vi "Basic_Acquire_Widefield.vi"() -> ()   [LabVIEW 2009]
uses:
  <vilib>/vision/Image Controls.llb/IMAQ Image.ctl
  <vilib>/userDefined/High Color/IMAQdx.ctl
  Widefield_globals.vi
  <vilib>/DAQmx/create/channels.llb/DAQmx Create Channel (DO-Digital Output).vi
  <vilib>/DAQmx/write.llb/DAQmx Write (Digital Bool 1Line 1Point).vi
  <vilib>/vision/NI_Vision_Development_Module.lvlib
  Program Files/National Instruments/LabVIEW 2009/resource/objmgr/imaqdx.rc
  <vilib>/vision/driver/NI_Vision_Acquisition_Software.lvlib
panel:
  out "RatioIm 2":u8[][](graph)
  out "frame number":i32
  out "IMAQ session":T1 caption="Session Out"
  out "frame times":i32[](array[numeric])
  out "error out":errorcluster
  out "LED settle":i32
  out "Control LED?":bool
  out "stim tag":string
  out "SF file":string
  out "One Bulb?":bool
  out "File Path":path
  out "SingleFrames":bool
  out "empty frame":dbl[][](array[numeric])
  out "Resolution":u32[](array[numeric])
  out "Experiment Sequence":dbl[][](array[numeric])
  out "settings":sgl[](array[numeric])
  out "Buff Img":T2
  out "COString":string
  in  "Offset (32768 default)":u32=32768
  in  "Contrast (600000 default)":u32=600000
  in  "Pause":bool=TRUE
  out "ExpOrderRefnum":refnum<file>
  out "Subframes":u32
  out "DCSAir":dbl[][](array[numeric])
  out "DCOdor":dbl[][](array[numeric])
  out "DCAir":dbl[][](array[numeric])
  out "TiffRefnum":refnum<file>
  out "Indices":i32[](array[numeric])
  out "Frames SAir":u32
  out "Odors:":u32
  out "StopAcq":bool
  in  "Stop":bool=TRUE
  out "Odor #":i32=50
  out "Repeats:":i32=1
  out "Repeat #":i32=1
  out "Frames Odor":u32
  out "Frames Air":u32
  out "Status":string
  out "Stimulus #":i32
  in  "start":bool=TRUE
  # "Filtered Ratio Image"
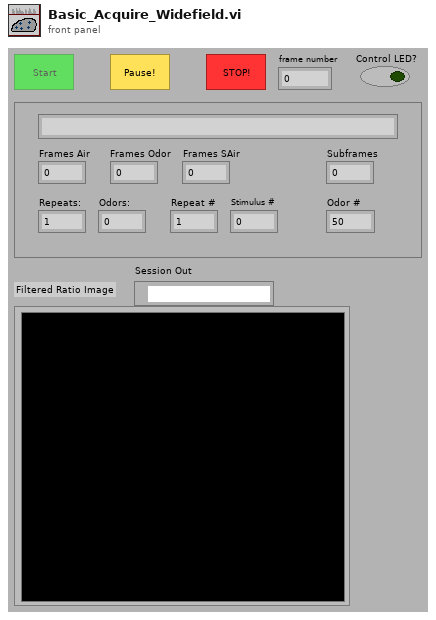
[diagram p1: front panel]
types:
  T1 = typedef "IMAQdx.ctl" = refnum<k21>
  T2 = typedef "IMAQ Image.ctl" = refnum<image>
  T3 = enum16{"open", "replace", "create", "open or create", "replace or create", "replace or create with confirmation"}
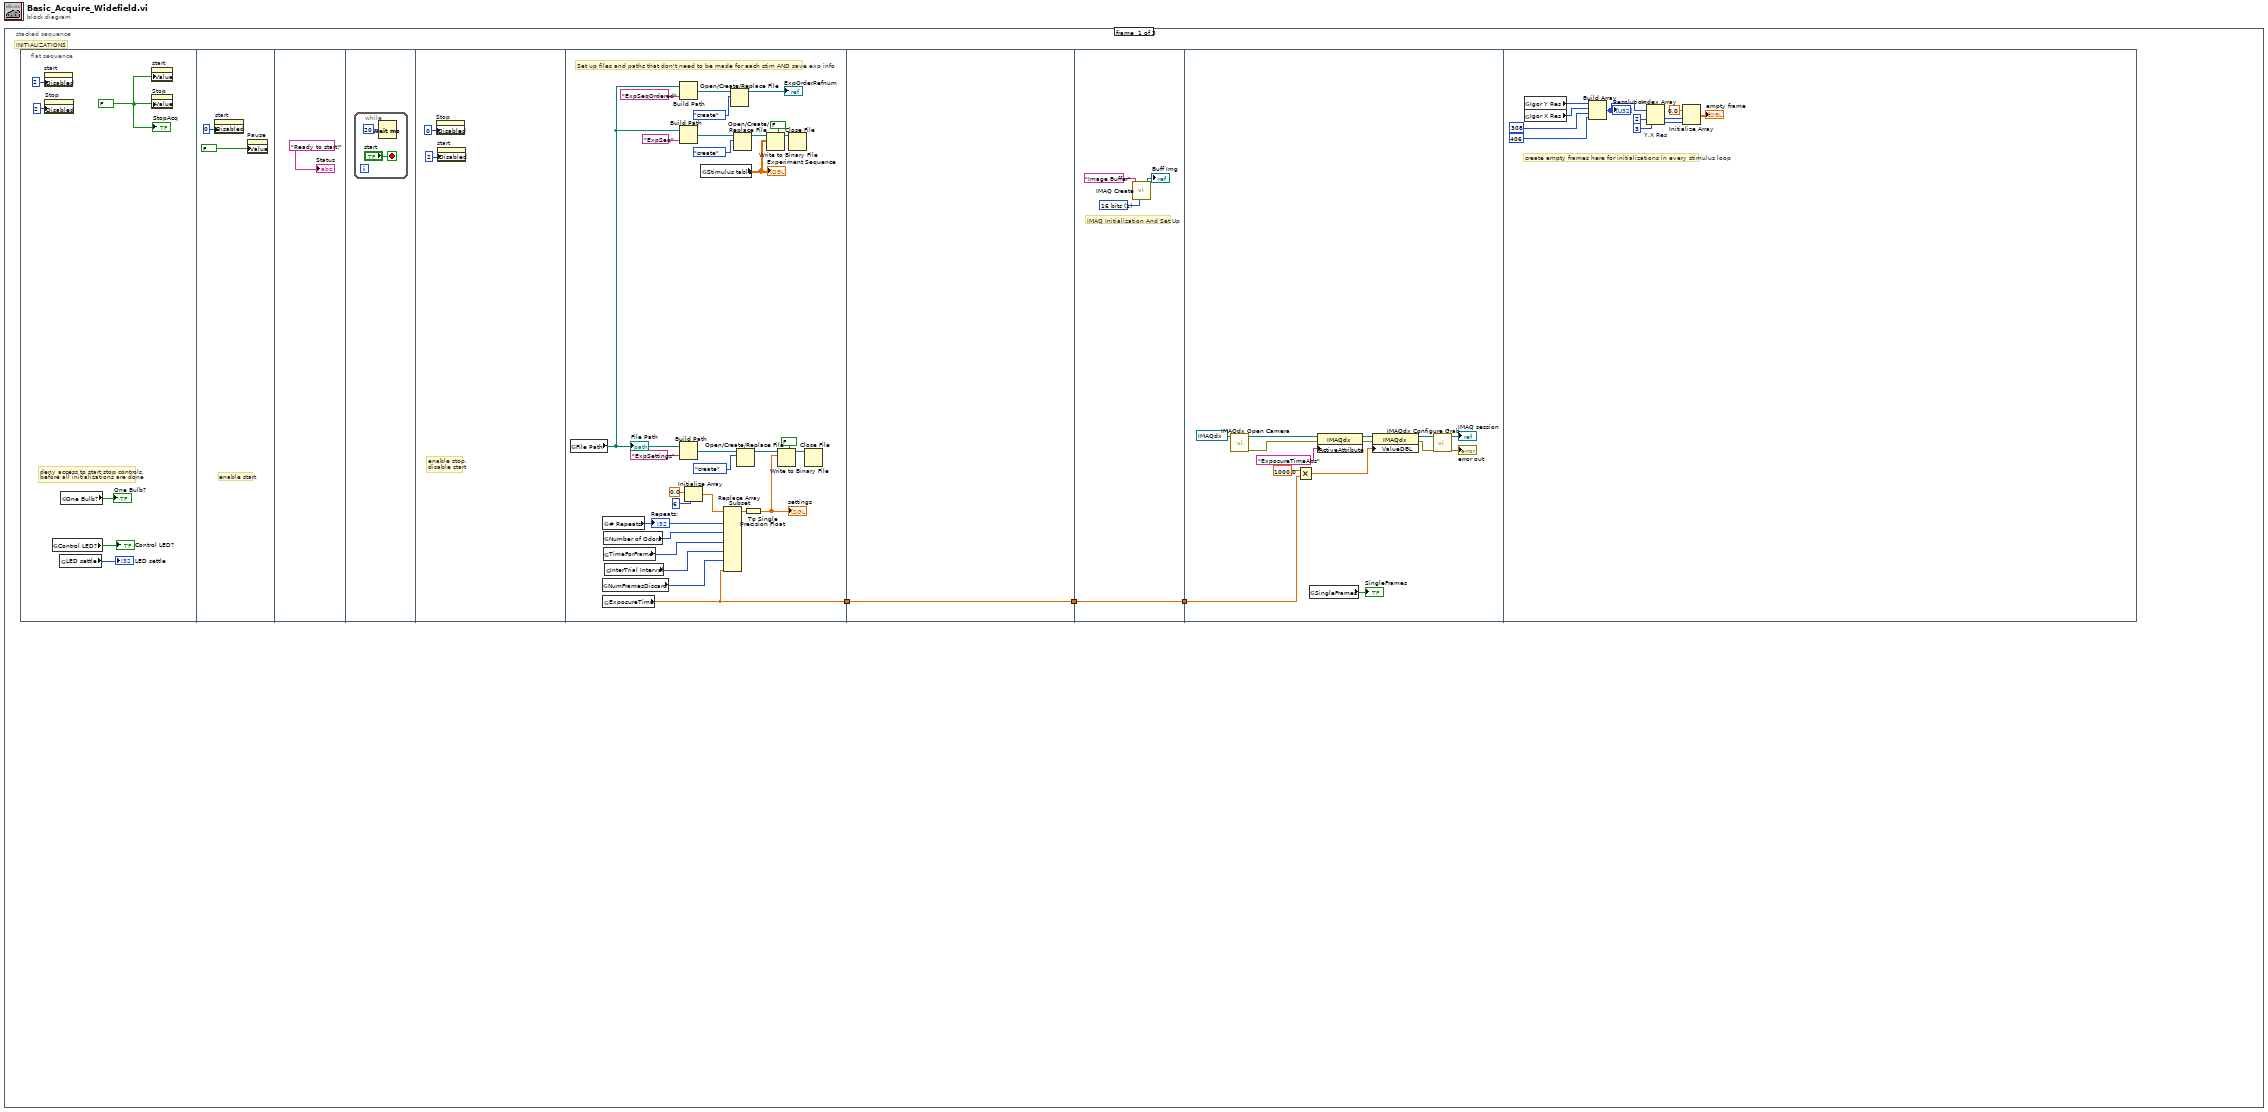
[diagram p0: block diagram]
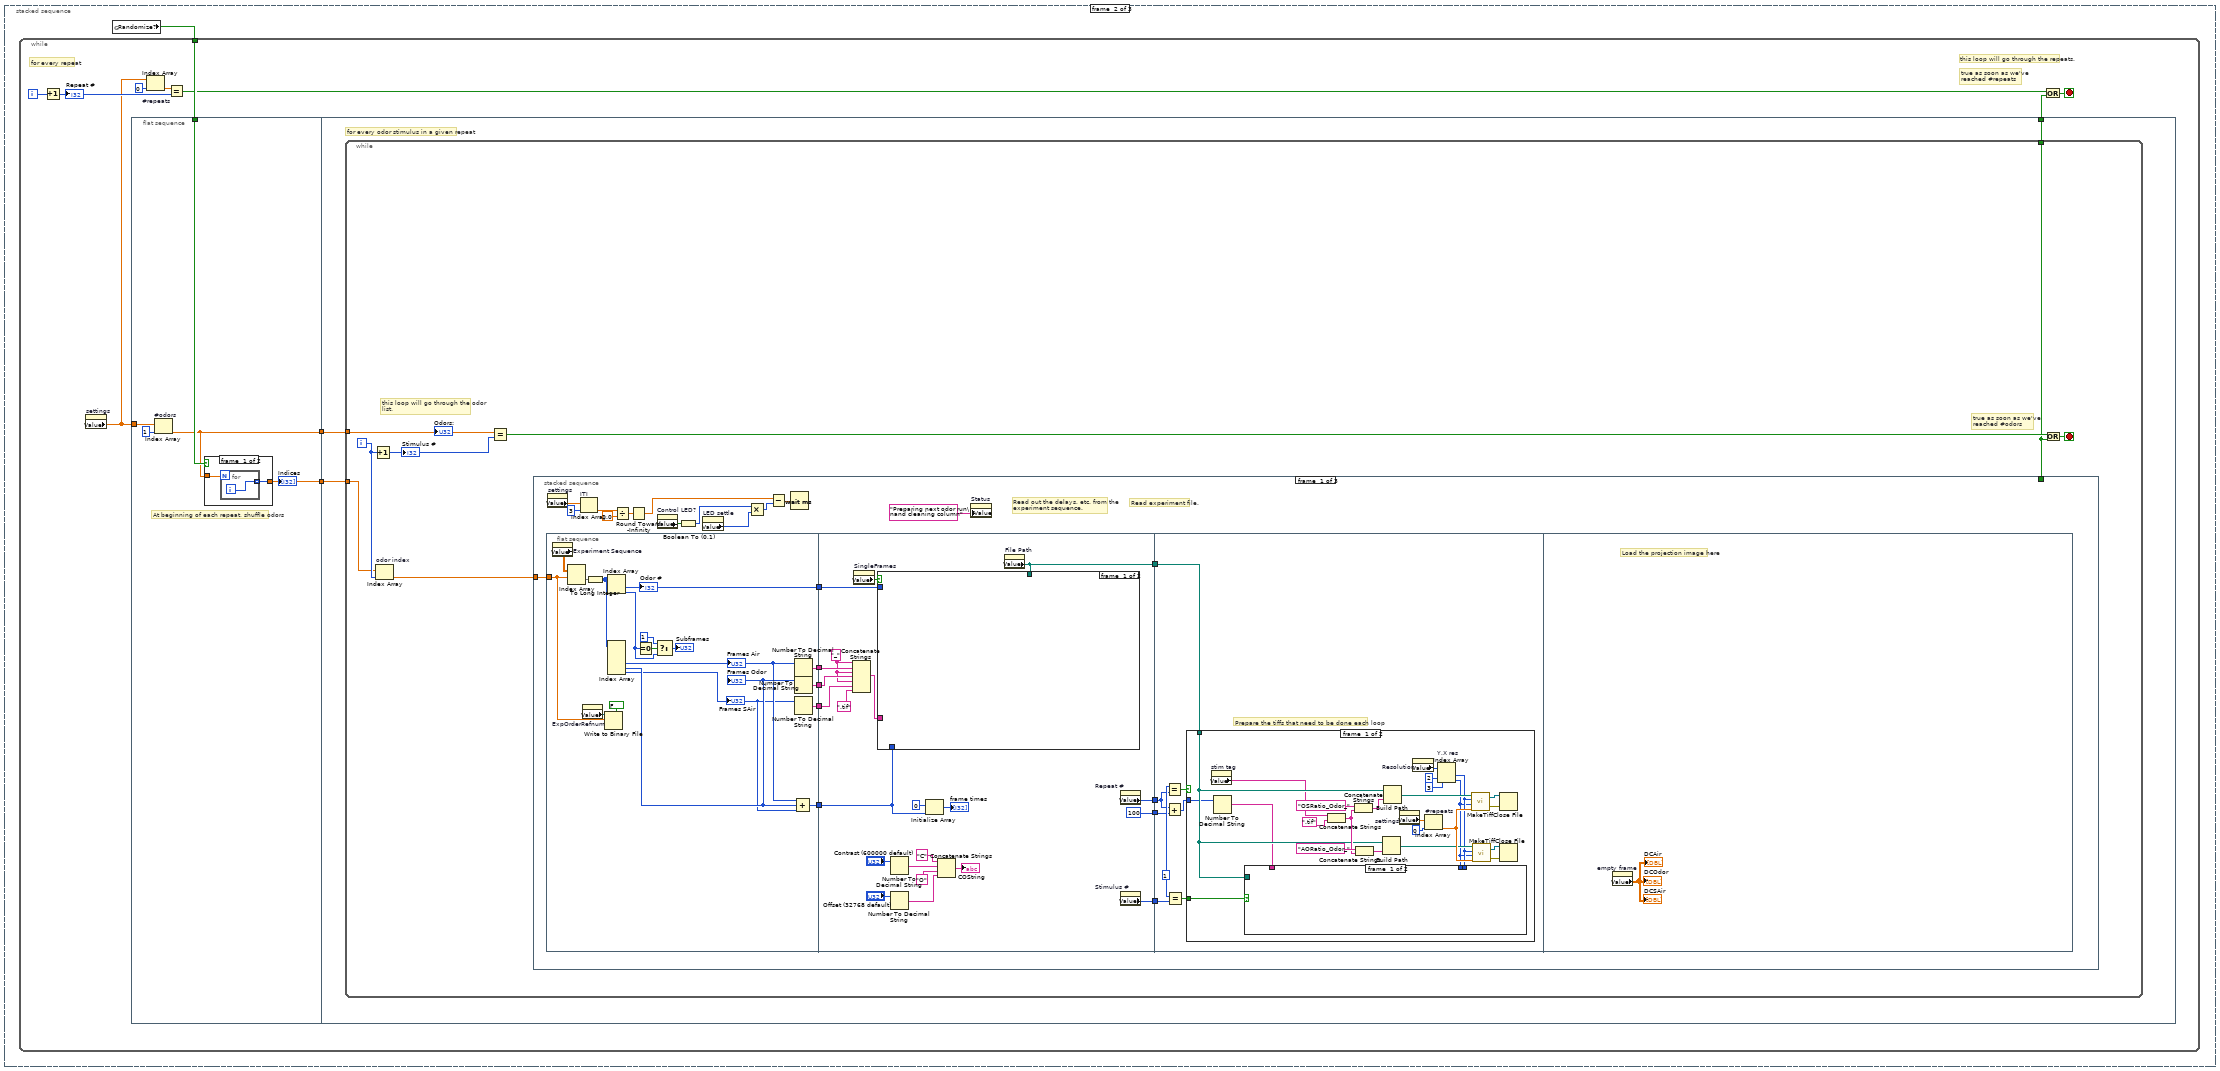
[diagram p2: hidden frame]
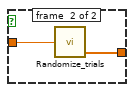
[diagram p3: hidden frame]
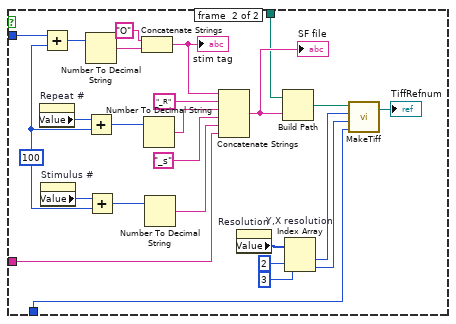
[diagram p4: hidden frame]
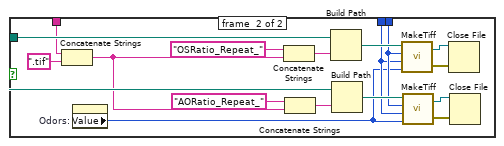
[diagram p5: hidden frame]
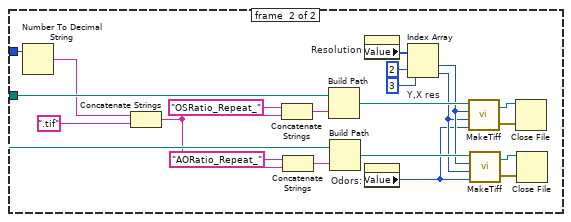
[diagram p7: hidden frame]
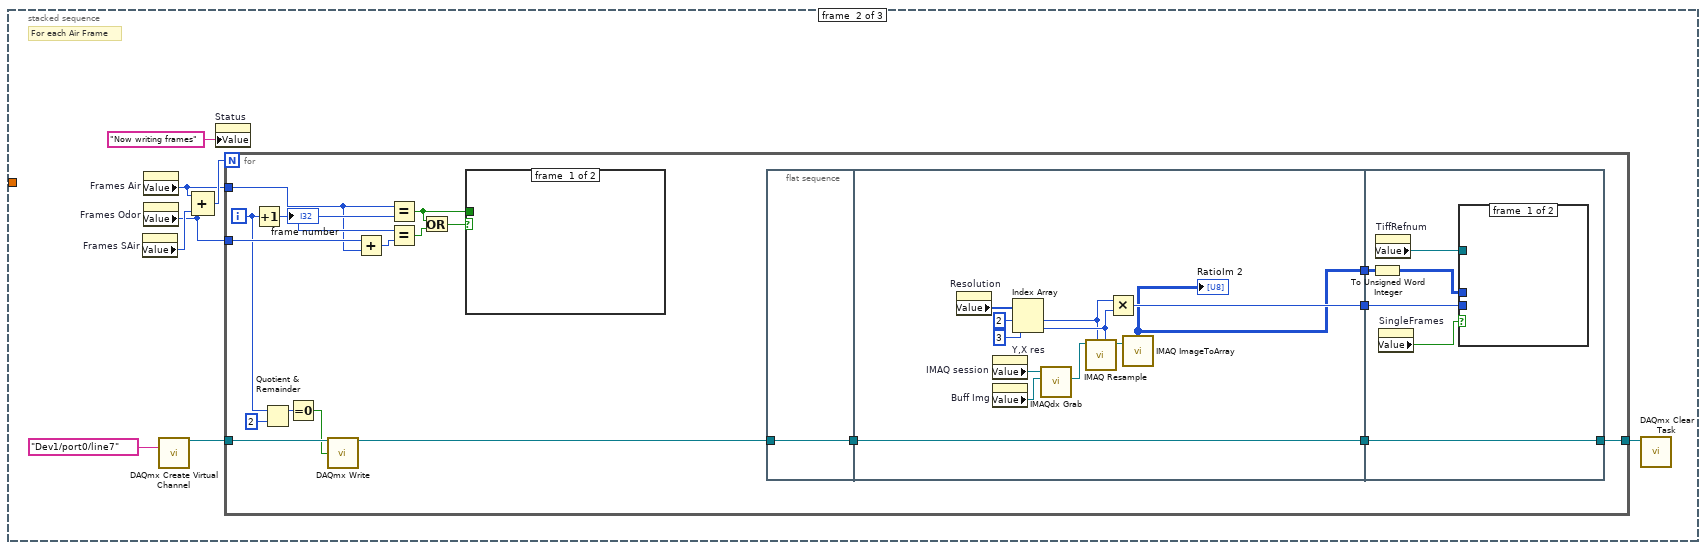
[diagram p8: hidden frame]
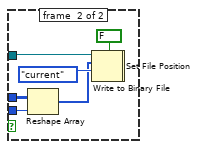
[diagram p9: hidden frame]
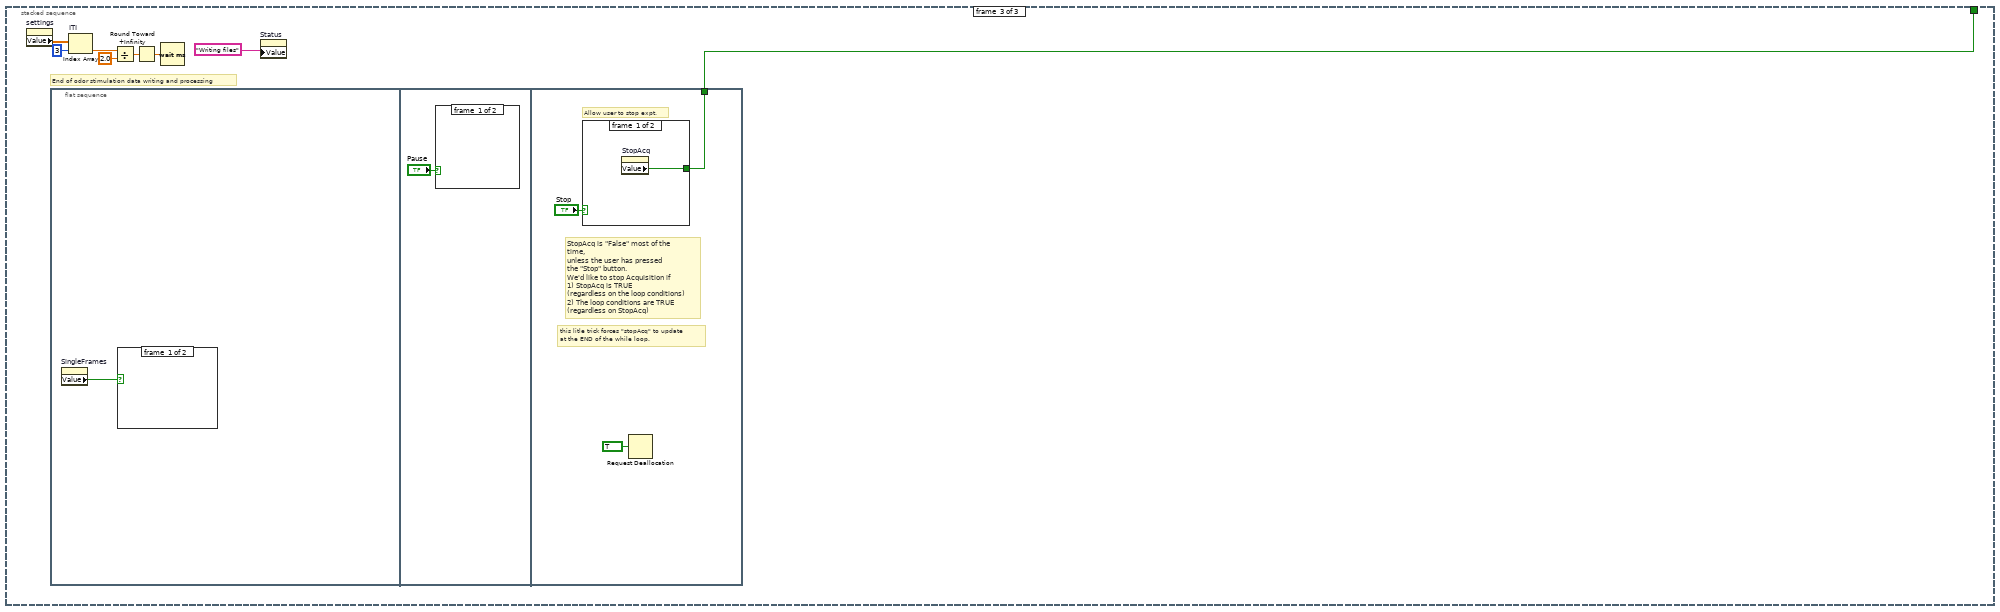
[diagram p12: hidden frame]
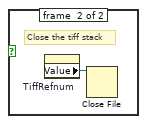
[diagram p13: hidden frame]
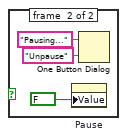
[diagram p14: hidden frame]
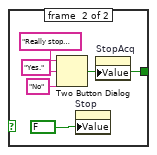
[diagram p15: hidden frame]
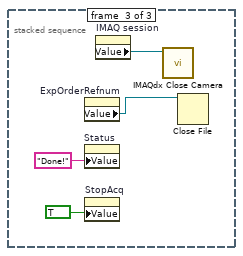
[diagram p16: hidden frame]
diagram:
  n1 = stacked-sequence {
    frame #0 {
      # "INITIALIZATIONS"
      n2 = flat-sequence {
        tunnel: [w18] -> w1
        tunnel: [w46] -> w2
        tunnel: w1 -> [w46]
        tunnel: [w47] -> w3
        tunnel: w2 -> [w47]
        tunnel: w3 -> [w57]
        frame #0 {
          w7 = FALSE ("Stop")
          # "deny access to start stop controls, \nbefore all initializations are done"
          n3 = property on="start" class="Boolean (strict)"("Disabled"=u8 2) -> ()  [unwired: 2 in, 2 out]
          n4 = property on="Stop" class="Bool (strict)"("Disabled"=u8 2) -> ()  [unwired: 2 in, 2 out]
          n5 = global read "Widefield_globals.vi" "Control LED?"() -> (→"Control LED?":bool)
          n6 = global read "Widefield_globals.vi" "LED settle"() -> (→"LED settle":i32)
          n7 = global read "Widefield_globals.vi" "One Bulb?"() -> (→"One Bulb?":bool)
          n8 = property on="start" class="Boolean (strict)"("Value"=w7) -> ()  [unwired: 2 in, 2 out]
          n9 = property on="Stop" class="Bool (strict)"("Value"=w7) -> ()  [unwired: 2 in, 2 out]
          "StopAcq" <- w7
        }
        frame #1 {
          # "enable start"
          n10 = property on="start" class="Boolean (strict)"("Disabled"=u8 0) -> ()  [unwired: 2 in, 2 out]
          n11 = property on="Pause" class="Bool (strict)"("Value"=FALSE ("Pause")) -> ()  [unwired: 2 in, 2 out]
        }
        frame #2 {
          "Status" <- "Ready to start!" ("Status")
        }
        frame #3 {
          n12 = while {
            stop <- "start" stop-if-true
            n13 = Wait (ms)(milliseconds to wait=u32 20) -> ()  [unwired: 1 out]
          }
        }
        frame #4 {
          # "enable stop,\ndisable start"
          n14 = property on="Stop" class="Bool (strict)"("Disabled"=u8 0) -> ()  [unwired: 2 in, 2 out]
          n15 = property on="start" class="Boolean (strict)"("Disabled"=u8 2) -> ()  [unwired: 2 in, 2 out]
        }
        frame #5 {
          # "Set up files and paths that don't need to be made for each stim AND save exp info"
          n16 = global read "Widefield_globals.vi" "File Path"() -> (w24:path)
          "File Path" <- w24
          n17 = global read "Widefield_globals.vi" "NumFramesDiscard"() -> (w19:i32)
          n18 = global read "Widefield_globals.vi" "# Repeats"() -> (w22:u16)
          "Repeats:" <- w22
          n19 = global read "Widefield_globals.vi" "ExposureTime"() -> (w18:dbl)
          n20 = global read "Widefield_globals.vi" "Number of Odors"() -> (w21:u32)
          n21 = global read "Widefield_globals.vi" "TimeForFrame"() -> (w17:u32)
          n22 = global read "Widefield_globals.vi" "InterTrial Interval"() -> (w20:i32)
          n23 = Build Path(base path=w24, name or relative path="ExpSeq" ("string")) -> (appended path=w37:path)
          n24 = Build Path(base path=w24, name or relative path="ExpSeqOrdered" ("string")) -> (appended path=w27:path)
          n25 = Build Path(base path=w24, name or relative path="ExpSettings" ("string")) -> (appended path=w35:path)
          n26 = Initialize Array(sgl 0.0 ("element"), 6 ("dimension size")) -> (w31:sgl[])
          n27 = global read "Widefield_globals.vi" "Stimulus table"() -> (w23:dbl[][])
          "Experiment Sequence" <- w23
          n28 = Replace Array Subset(array=w31, new element #1=w22, new element #2=w21, new element #3=w17, new element #4=w20, new element #5=w19, new element #6=w18) -> (w30:sgl[])  [unwired: 6 in]
          n29 = Open/Create/Replace File(file path (use dialog)=w27, operation (0:open)=T3."create") -> (refnum out=→"ExpOrderRefnum":refnum<file>)  [unwired: 1 in, 5 out]
          n30 = Open/Create/Replace File(file path (use dialog)=w37, operation (0:open)=T3."create") -> (refnum out=w44:refnum<file>)  [unwired: 1 in, 5 out]
          n31 = Open/Create/Replace File(file path (use dialog)=w35, operation (0:open)=T3."create") -> (refnum out=w43:refnum<file>)  [unwired: 1 in, 5 out]
          n32 = To Single Precision Float(number=w30) -> (single precision float=w29:sgl[])
          "settings" <- w29
          n33 = Write to Binary File(file (use dialog)=w44, data=w23, 5:FALSE ("prepend array or string size? (T)")) -> (refnum out=w45:refnum<file>)  [unwired: 1 in, 4 out]
          n34 = Write to Binary File(file (use dialog)=w43, data=w29, 5:FALSE ("prepend array or string size? (T)")) -> (refnum out=w28:refnum<file>)  [unwired: 1 in, 4 out]
          n35 = Close File(refnum=w45) -> ()  [unwired: 1 in, 2 out]
          n36 = Close File(refnum=w28) -> ()  [unwired: 1 in, 2 out]
        }
        frame #6 {
        }
        frame #7 {
          w50 = u32 1 items=["8 bits", "16 bits", "Float", "Complex", "RGB", "HSL"] ("Image Type")
          # "IMAQ Initialization And Set Up"
          n37 = call "IMAQ Create"("Image Name"="Image Buffer", "Image Type"=w50) -> ("New Image"=→"Buff Img":T2)  [unwired: 2 in, 2 out]
        }
        frame #8 {
          n38 = call <vilib>:"IMAQdx Open Camera.vi"("Session In"=T1 "cam0") -> ("error out"=w60:errorcluster, "Session Out"=w59:T1)  [unwired: 2 in, 7 out]
          n39 = Multiply(x=1000.0 ("y"), y=w57) -> (x*y=w53:dbl)
          n40 = global read "Widefield_globals.vi" "SingleFrames"() -> (→"SingleFrames":bool)
          n41 = property class="IMAQdx"(reference=w59, error in=w60, "ActiveAttribute"="ExposureTimeAbs" ("Camera Attribute")) -> (reference out=w54:T1, error out=w55:errorcluster)
          n42 = property class="IMAQdx"(reference=w54, error in=w55, "ValueDBL"=w53) -> (reference out=w62:T1, error out=w58:errorcluster)
          n43 = call <vilib>:"IMAQdx Configure Grab.vi"("error in"=w58, "Session In"=w62) -> ("error out"=→"error out":errorcluster, "Session Out"=→"IMAQ session":T1)  [unwired: 8 out]
        }
        frame #9 {
          # "create empty frames here for initializations in every stimulus loop"
          n44 = global read "Widefield_globals.vi" "Igor Y Res"() -> (w69:u32)
          n45 = global read "Widefield_globals.vi" "Igor X Res"() -> (w68:u32)
          n46 = Build Array(w69, w68, u32 308 ("Y Res"), u32 406 ("X Res")) -> (w67:u32[])
          "Resolution" <- w67
          n47 = Index Array "Y,X Res"(array=w67, index #1=2 ("index"), index #2=3 ("index")) -> (element #1=w75:u32, element #2=w74:u32)
          n48 = Initialize Array(0.0 ("element"), w75, w74) -> (→"empty frame":dbl[][])
        }
      }
    }
    frame #1 {
      n49 = global read "Widefield_globals.vi" "Randomize?"() -> (w76:bool)
      n50 = while {
        tunnel: w76 -> [w85]
        i -> [w80]
        stop <- w87 stop-if-true
        # "for every repeat"
        # "this loop will go through the repeats."
        # "true as soon as we've\nreached #repeats"
        n51 = Increment(x=w80) -> (x+1=w86:i32)
        "Repeat #" <- w86
        n52 = property on="settings" class="Arr (strict)"() -> ("Value"=w82:sgl[])  [unwired: 2 in, 2 out]
        n53 = flat-sequence {
          tunnel: w82 -> [w92]
          tunnel: w85 -> [w90]
          tunnel: [w89] -> w84
          tunnel: [w88] -> w83
          tunnel: w84 -> [w100]
          tunnel: w83 -> [w99]
          tunnel: [w98] -> w78
          frame #0 {
            # "At beginning of each repeat, shuffle odors"
            n54 = Index Array "#odors"(array=w92, index=1) -> (element=w89:sgl)
            n55 = case shown="True" w90 {
              tunnel: [w93 w97] -> w88
              tunnel: w89 -> [w94 w96]
              frame #0 {
                n56 = for {
                  N: w94 -> [_]
                  tunnel: [w95] -> w93 mode=indexing
                  i -> [w95]
                }
              }
              frame #1 {
                n57 = call "Randomize_trials.vi"("ArraySize"=w96) -> ("Randomized"=w97:dbl[])  [unwired: 2 in]
              }
            }
            "Indices" <- w88
          }
          frame #1 {
            # "for every odor stimulus in a given repeat"
            n58 = while {
              tunnel: w100 -> [w107]
              tunnel: w99 -> [w104]
              tunnel: [w102] -> w98
              i -> [w106]
              stop <- w108 stop-if-true
              # "this loop will go through the odor\nlist."
              # "true as soon as we've\nreached #odors"
              n59 = Increment(x=w106) -> (x+1=w101:i32)
              "Stimulus #" <- w101
              n60 = Index Array "odor index"(array=w104, index=w106) -> (element=w105:dbl)
              n61 = Equal?(x=w107, y=w101) -> (x = y?=w103:bool)
              n62 = stacked-sequence {
                tunnel: w105 -> [w130 _ _]
                tunnel: [_ _ w332] -> w102
                frame #0 {
                  # "Read experiment file."
                  # "Read out the delays, etc. from the\nexperiment sequence."
                  n63 = flat-sequence {
                    tunnel: [w146] -> w129
                    tunnel: [w145] -> w128
                    tunnel: [w144] -> w127
                    tunnel: [w143] -> w126
                    tunnel: [w142] -> w125
                    tunnel: w130 -> [w134]
                    tunnel: [w162] -> w124
                    tunnel: [w163] -> w123
                    tunnel: [w161] -> w122
                    tunnel: w125 -> [w151]
                    tunnel: w126 -> [w157]
                    tunnel: w127 -> [w158]
                    tunnel: w128 -> [w159]
                    tunnel: w129 -> [w160]
                    tunnel: [100 ("y")] -> w114
                    tunnel: w124 -> [w197]
                    tunnel: w123 -> [w202]
                    tunnel: w122 -> [w201]
                    tunnel: w114 -> [w198]
                    frame #0 {
                      n64 = property on="Experiment Sequence" class="Arr (strict)"() -> ("Value"=w141:dbl[][])  [unwired: 2 in, 2 out]
                      n65 = Index Array(array=w141, index (row)=w134) -> (element=w140:dbl[])  [unwired: 1 in]
                      n66 = property on="ExpOrderRefnum" class="Ref (strict)"() -> ("Value"=w147:refnum<file>)  [unwired: 2 in, 2 out]
                      n67 = To Long Integer(number=w140) -> (32bit integer=w136:i32[])
                      n68 = Write to Binary File(file (use dialog)=w147, data=w134, 5:FALSE ("prepend array or string size? (T)")) -> ()  [unwired: 1 in, 5 out]
                      n69 = Index Array(array=w136) -> (element #1=w143:i32, element #2=w133:i32)  [unwired: 2 in]
                      "Odor #" <- w143
                      n70 = Index Array(array=w136) -> (element #3=w132:i32, element #4=w135:i32, element #5=w131:i32)  [unwired: 5 in, 2 out]
                      "Frames Air" <- w132
                      "Frames Odor" <- w135
                      "Frames SAir" <- w131
                      n71 = Equal To 0?(x=w133) -> (x = 0?=w139:bool)
                      n72 = Select(t=1, s=w139, f=w133) -> (s? t:f=→"Subframes":i32)
                      n73 = Number To Decimal String(number=w132) -> (decimal integer string=w146:string)  [unwired: 1 out]
                      n74 = Number To Decimal String(number=w135) -> (decimal integer string=w145:string)  [unwired: 1 out]
                      n75 = Number To Decimal String(number=w131) -> (decimal integer string=w144:string)  [unwired: 1 out]
                      n76 = Compound Arithmetic op=ADD(w132, w135, w131) -> (w142:i32)
                    }
                    frame #1 {
                      w154 = "_" ("string")
                      n77 = Concatenate Strings(w154, w160, w154, w159, w154, w158, ".tif" ("string")) -> (w155:string)
                      n78 = property on="SingleFrames" class="Bool (strict)"() -> ("Value"=w156:bool)  [unwired: 2 in, 2 out]
                      n79 = Number To Decimal String(number="Contrast (600000 default)") -> (decimal integer string=w166:string)  [unwired: 1 out]
                      n80 = Number To Decimal String(number="Offset (32768 default)") -> (decimal integer string=w165:string)  [unwired: 1 out]
                      n81 = Initialize Array(0 ("element"), w151) -> (→"frame times":i32[])
                      n82 = Concatenate Strings("C" ("string"), w166, "O" ("string"), w165) -> (→"COString":string)
                      n83 = property on="File Path" class="Path"() -> ("Value"=w163:path)  [unwired: 2 in, 2 out]
                      n84 = case shown="True" w156 {
                        tunnel: w157 -> [_ w190]
                        tunnel: w163 -> [_ w178]
                        tunnel: w155 -> [_ w171]
                        tunnel: w151 -> [_ w188]
                        frame #0 {
                        }
                        frame #1 {
                          w189 = 100 ("y")
                          n85 = property on="Repeat #" class="DigNum (strict)"() -> ("Value"=w181:i32)  [unwired: 2 in, 2 out]
                          n86 = property on="Stimulus #" class="DigNum (strict)"() -> ("Value"=w174:i32)  [unwired: 2 in, 2 out]
                          n87 = Add(x=w190, y=w189) -> (x+y=w194:i32)
                          n88 = Number To Decimal String(number=w194) -> (decimal integer string=w176:string)  [unwired: 1 out]
                          n89 = Add(x=w181, y=w189) -> (x+y=w195:i32)
                          n90 = Add(x=w174, y=w189) -> (x+y=w191:i32)
                          n91 = Concatenate Strings("O" ("string"), w176) -> (w175:string)
                          "stim tag" <- w175
                          n92 = Number To Decimal String(number=w195) -> (decimal integer string=w193:string)  [unwired: 1 out]
                          n93 = Number To Decimal String(number=w191) -> (decimal integer string=w172:string)  [unwired: 1 out]
                          n94 = Concatenate Strings(w175, "_R" ("string"), w193, "_s" ("string"), w172, w171) -> (w180:string)
                          "SF file" <- w180
                          n95 = property on="Resolution" class="Arr (strict)"() -> ("Value"=w186:u32[])  [unwired: 2 in, 2 out]
                          n96 = Build Path(base path=w178, name or relative path=w180) -> (appended path=w179:path)
                          n97 = Index Array "Y,X resolution"(array=w186, index #1=2 ("index"), index #2=3 ("index")) -> (element #1=w183:u32, element #2=w182:u32)
                          n98 = call "MakeTiff.vi"("z"=w188, "X"=w182, "Y"=w183, "file path"=w179) -> ("refnum tif"=→"TiffRefnum":refnum<file>)  [unwired: 1 out]
                        }
                      }
                      n99 = property on="Repeat #" class="DigNum (strict)"() -> ("Value"=w162:i32)  [unwired: 2 in, 2 out]
                      n100 = property on="Stimulus #" class="DigNum (strict)"() -> ("Value"=w161:i32)  [unwired: 2 in, 2 out]
                    }
                    frame #2 {
                      w200 = 1 ("x")
                      # "Prepare the tiffs that need to be done each loop"
                      n101 = Equal?(x=w200, y=w197) -> (x = y?=w203:bool)
                      n102 = Add(x=w197, y=w198) -> (x+y=w196:i32)
                      n103 = Equal?(x=w200, y=w201) -> (x = y?=w199:bool)
                      n104 = case shown="False" w203 {
                        tunnel: w202 -> [w211 w248]
                        tunnel: w196 -> [w207 w247]
                        tunnel: w199 -> [w206 w246]
                        frame #0 {
                          n105 = property on="stim tag" class="Str"() -> ("Value"=w205:string)  [unwired: 2 in, 2 out]
                          n106 = Number To Decimal String(number=w207) -> (decimal integer string=w208:string)  [unwired: 1 out]
                          n107 = Concatenate Strings(w205, ".tif" ("string")) -> (w220:string)
                          n108 = Concatenate Strings("OSRatio_Odor_" ("string"), w220) -> (w222:string)
                          n109 = Concatenate Strings("AORatio_Odor_" ("string"), w220) -> (w219:string)
                          n110 = Build Path(base path=w211, name or relative path=w219) -> (appended path=w212:path)
                          n111 = Build Path(base path=w211, name or relative path=w222) -> (appended path=w224:path)
                          n112 = property on="settings" class="Arr (strict)"() -> ("Value"=w214:sgl[])  [unwired: 2 in, 2 out]
                          n113 = property on="Resolution" class="Arr (strict)"() -> ("Value"=w218:u32[])  [unwired: 2 in, 2 out]
                          n114 = Index Array "#repeats"(array=w214, index=0) -> (element=w213:sgl)
                          n115 = Index Array "Y,X res"(array=w218, index #1=2 ("index"), index #2=3 ("index")) -> (element #1=w210:u32, element #2=w209:u32)
                          n116 = case shown="True" w206 {
                            tunnel: w211 -> [_ w235]
                            tunnel: w210 -> [_ w234]
                            tunnel: w209 -> [_ w233]
                            tunnel: w208 -> [_ w231]
                            frame #0 {
                            }
                            frame #1 {
                              n117 = Concatenate Strings(w231, ".tif" ("string")) -> (w232:string)
                              n118 = property on="Odors:" class="DigNum (strict)"() -> ("Value"=w230:u32)  [unwired: 2 in, 2 out]
                              n119 = Concatenate Strings("OSRatio_Repeat_" ("string"), w232) -> (w245:string)
                              n120 = Concatenate Strings("AORatio_Repeat_" ("string"), w232) -> (w237:string)
                              n121 = Build Path(base path=w235, name or relative path=w245) -> (appended path=w236:path)
                              n122 = Build Path(base path=w235, name or relative path=w237) -> (appended path=w239:path)
                              n123 = call "MakeTiff.vi"("z"=w230, "X"=w233, "Y"=w234, "file path"=w236) -> ("error out"=w243:errorcluster, "refnum tif"=w242:refnum<file>)
                              n124 = call "MakeTiff.vi"("z"=w230, "X"=w233, "Y"=w234, "file path"=w239) -> ("error out"=w240:errorcluster, "refnum tif"=w241:refnum<file>)
                              n125 = Close File(refnum=w242, error in=w243) -> ()  [unwired: 2 out]
                              n126 = Close File(refnum=w241, error in=w240) -> ()  [unwired: 2 out]
                            }
                          }
                          n127 = call "MakeTiff.vi"("z"=w213, "X"=w209, "Y"=w210, "file path"=w224) -> ("error out"=w225:errorcluster, "refnum tif"=w226:refnum<file>)
                          n128 = call "MakeTiff.vi"("z"=w213, "X"=w209, "Y"=w210, "file path"=w212) -> ("error out"=w227:errorcluster, "refnum tif"=w228:refnum<file>)
                          n129 = Close File(refnum=w226, error in=w225) -> ()  [unwired: 2 out]
                          n130 = Close File(refnum=w228, error in=w227) -> ()  [unwired: 2 out]
                        }
                        frame #1 {
                          n131 = case shown="True" w246 {
                            tunnel: w248 -> [_ w256]
                            tunnel: w247 -> [_ w251]
                            frame #0 {
                            }
                            frame #1 {
                              n132 = Number To Decimal String(number=w251) -> (decimal integer string=w252:string)  [unwired: 1 out]
                              n133 = Concatenate Strings(w252, ".tif" ("string")) -> (w253:string)
                              n134 = Concatenate Strings("OSRatio_Repeat_" ("string"), w253) -> (w266:string)
                              n135 = Concatenate Strings("AORatio_Repeat_" ("string"), w253) -> (w258:string)
                              n136 = Build Path(base path=w256, name or relative path=w266) -> (appended path=w257:path)
                              n137 = Build Path(base path=w256, name or relative path=w258) -> (appended path=w260:path)
                              n138 = property on="Resolution" class="Arr (strict)"() -> ("Value"=w269:u32[])  [unwired: 2 in, 2 out]
                              n139 = property on="Odors:" class="DigNum (strict)"() -> ("Value"=w250:u32)  [unwired: 2 in, 2 out]
                              n140 = Index Array "Y,X res"(array=w269, index #1=2 ("index"), index #2=3 ("index")) -> (element #1=w255:u32, element #2=w254:u32)
                              n141 = call "MakeTiff.vi"("z"=w250, "X"=w254, "Y"=w255, "file path"=w257) -> ("error out"=w264:errorcluster, "refnum tif"=w263:refnum<file>)
                              n142 = call "MakeTiff.vi"("z"=w250, "X"=w254, "Y"=w255, "file path"=w260) -> ("error out"=w261:errorcluster, "refnum tif"=w262:refnum<file>)
                              n143 = Close File(refnum=w263, error in=w264) -> ()  [unwired: 2 out]
                              n144 = Close File(refnum=w262, error in=w261) -> ()  [unwired: 2 out]
                            }
                          }
                        }
                      }
                    }
                    frame #3 {
                      # "Load the projection image here"
                      n145 = property on="empty frame" class="Arr (strict)"() -> ("Value"=→"DCAir" →"DCOdor" →"DCSAir":dbl[][])  [unwired: 2 in, 2 out]
                    }
                  }
                  n146 = property on="settings" class="Arr (strict)"() -> ("Value"=w121:sgl[])  [unwired: 2 in, 2 out]
                  n147 = Index Array "ITI"(array=w121, index=3) -> (element=w119:sgl)
                  n148 = Divide(x=w119, y=sgl 2.0) -> (x/y=w117:sgl)
                  n149 = Round Toward -Infinity(1:w117) -> (0:w116:sgl)
                  n150 = property on="Control LED?" class="Bool (strict)"() -> ("Value"=w112:bool)  [unwired: 2 in, 2 out]
                  n151 = Boolean To (0,1)(Boolean=w112) -> (0, 1=w110:i16)
                  n152 = property on="LED settle" class="DigNum (strict)"() -> ("Value"=w109:i32)  [unwired: 2 in, 2 out]
                  n153 = Multiply(x=w110, y=w109) -> (x*y=w111:i32)
                  n154 = Subtract(x=w116, y=w111) -> (x-y=w113:sgl)
                  n155 = Wait (ms)(milliseconds to wait=w113) -> ()  [unwired: 1 out]
                  n156 = property on="Status" class="Str"("Value"="Preparing next odor run\nand cleaning column" ("Status")) -> ()  [unwired: 2 in, 2 out]
                }
                frame #1 {
                  # "For each Air Frame"
                  n157 = property on="Frames SAir" class="DigNum (strict)"() -> ("Value"=w277:u32)  [unwired: 2 in, 2 out]
                  n158 = property on="Frames Air" class="DigNum (strict)"() -> ("Value"=w275:u32)  [unwired: 2 in, 2 out]
                  n159 = property on="Frames Odor" class="DigNum (strict)"() -> ("Value"=w274:u32)  [unwired: 2 in, 2 out]
                  n160 = call-poly <vilib>:"DAQmx Create Virtual Channel.vi"("lines"=tag "Dev1/port0/line7") -> ("task out"=w272:refnum<k21>)  [unwired: 13 in, 1 out]
                  n161 = Compound Arithmetic op=ADD(w275, w274, w277) -> (w276:u32)
                  n162 = property on="Status" class="Str"("Value"="Now writing frames" ("String")) -> ()  [unwired: 2 in, 2 out]
                  n163 = for {
                    N: w276 -> [_]
                    tunnel: w275 -> [w291]
                    tunnel: w274 -> [w293]
                    tunnel: w272 -> [w284]
                    tunnel: [w279] -> w271
                    i -> [w287]
                    n164 = Increment(x=w287) -> (x+1=w294:i32)
                    "frame number" <- w294
                    n165 = Quotient & Remainder(x=w287, y=2) -> (x-y*floor(x/y)=w285:i32)  [unwired: 1 out]
                    n166 = Equal To 0?(x=w285) -> (x = 0?=w283:bool)
                    n167 = call-poly <vilib>:"DAQmx Write.vi"("task/channels in"=w284, "data"=w283) -> ("task out"=w280:refnum<k21>)  [unwired: 11 in, 2 out]
                    n168 = Add(x=w293, y=w291) -> (x+y=w292:u32)
                    n169 = Equal?(x=w291, y=w294) -> (x = y?=w288:bool)
                    n170 = Equal?(x=w294, y=w292) -> (x = y?=w289:bool)
                    n171 = Or(x=w288, y=w289) -> (x .or. y?=w290:bool)
                    n172 = case shown="True" w290 {
                      tunnel: w288 -> [_ w324]
                      frame #0 {
                      }
                      frame #1 {
                        n173 = case shown="True" w324 {
                          frame #0 {
                          }
                          frame #1 {
                          }
                        }
                      }
                    }
                    n174 = flat-sequence {
                      tunnel: [w297] -> w281
                      tunnel: w280 -> [w297]
                      tunnel: [w309] -> w296
                      tunnel: [w299] -> w295
                      tunnel: [w298] -> w282
                      tunnel: w281 -> [w298]
                      tunnel: w296 -> [w315]
                      tunnel: w295 -> [w314]
                      tunnel: w282 -> [w310]
                      tunnel: [w310] -> w279
                      frame #0 {
                      }
                      frame #1 {
                        n175 = property on="Resolution" class="Arr (strict)"() -> ("Value"=w306:u32[])  [unwired: 2 in, 2 out]
                        n176 = property on="IMAQ session" class="IMAQdx (strict)"() -> ("Value"=w304:refnum<k21>)  [unwired: 2 in, 2 out]
                        n177 = property on="Buff Img" class="IMAQImage (strict)"() -> ("Value"=w305:refnum<image>)  [unwired: 2 in, 2 out]
                        n178 = Index Array "Y,X res"(array=w306, index #1=2 ("index"), index #2=3 ("index")) -> (element #1=w302:u32, element #2=w303:u32)
                        n179 = call <vilib>:"IMAQdx Grab.vi"("Image In"=w305, "Session In"=w304) -> ("Image Out"=w301:T2)  [unwired: 2 in, 7 out]
                        n180 = call "IMAQ Resample"("X Resolution"=w303, "Y Resolution"=w302, "Image Src"=w301) -> ("Image Dst Out"=w300:T2)  [unwired: 4 in, 4 out]
                        n181 = Multiply(x=w302, y=w303) -> (x*y=w309:u32)
                        n182 = call "IMAQ ImageToArray"("Image"=w300) -> ("Image Pixels (U8)"=w299:u8[][])  [unwired: 2 in, 5 out]
                        "RatioIm 2" <- w299
                      }
                      frame #2 {
                        n183 = To Unsigned Word Integer(number=w314) -> (unsigned 16bit integer=w313:u16[][])
                        n184 = property on="TiffRefnum" class="Ref (strict)"() -> ("Value"=w312:refnum<file>)  [unwired: 2 in, 2 out]
                        n185 = property on="SingleFrames" class="Bool (strict)"() -> ("Value"=w311:bool)  [unwired: 2 in, 2 out]
                        n186 = case shown="True" w311 {
                          tunnel: w315 -> [_ w322]
                          tunnel: w313 -> [_ w320]
                          tunnel: w312 -> [_ w319]
                          frame #0 {
                          }
                          frame #1 {
                            n187 = Reshape Array(w320, w322) -> (w321:u16[])
                            n188 = Set File Position(refnum=w319, from (0:start)=enum16{"start", "end", "current"}."current" ("pos mode (0:2)")) -> (refnum out=w318:refnum<file>, error out=w317:errorcluster)  [unwired: 1 in, 1 out]
                            n189 = Write to Binary File(file (use dialog)=w318, data=w321, error in=w317, 5:FALSE ("prepend array or string size? (T)")) -> ()  [unwired: 5 out]
                          }
                        }
                      }
                    }
                  }
                  n190 = call <vilib>:"DAQmx Clear Task.vi"("task in"=w271) -> ()  [unwired: 14 in, 1 out]
                }
                frame #2 {
                  # "End of odor stimulation data writing and processing"
                  n191 = property on="settings" class="Arr (strict)"() -> ("Value"=w331:sgl[])  [unwired: 2 in, 2 out]
                  n192 = flat-sequence {
                    tunnel: [w340] -> w332
                    frame #0 {
                      n193 = property on="SingleFrames" class="Bool (strict)"() -> ("Value"=w333:bool)  [unwired: 2 in, 2 out]
                      n194 = case shown="True" w333 {
                        frame #0 {
                        }
                        frame #1 {
                          # "Close the tiff stack"
                          n195 = property on="TiffRefnum" class="Ref (strict)"() -> ("Value"=w334:refnum<file>)  [unwired: 2 in, 2 out]
                          n196 = Close File(refnum=w334) -> ()  [unwired: 1 in, 2 out]
                        }
                      }
                    }
                    frame #1 {
                      n197 = case shown="True" "Pause" {
                        frame #0 {
                        }
                        frame #1 {
                          n198 = property on="Pause" class="Bool (strict)"("Value"=FALSE ("Pause")) -> ()  [unwired: 2 in, 2 out]
                          n199 = One Button Dialog(message="Pausing...", button name ("OK")="Unpause") -> ()  [unwired: 1 out]
                        }
                      }
                    }
                    frame #2 {
                      # "this litle trick forces \"stopAcq\" to update\nat the END of the while loop."
                      # "StopAcq is \"False\" most of the time, \nunless the user has pressed\nthe \"Stop\" button.\nWe'd like to stop Acquisition if\n1) StopAcq is TRUE \n(regardless on the loop conditions)\n2) The loop conditions are TRUE \n(regardless on StopAcq)"
                      # "Allow user to stop expt."
                      n200 = case shown="True" "Stop" {
                        tunnel: [w342 w343] -> w340
                        frame #0 {
                          n201 = property on="StopAcq" class="Bool (strict)"() -> ("Value"=w342:bool)  [unwired: 2 in, 2 out]
                        }
                        frame #1 {
                          n202 = Two Button Dialog(message="Really stop acquisition after this stimulus?", 1:"No" ("F button name (\"Cancel\")"), 2:"Yes." ("T button name (\"OK\")")) -> (T button?=w343:bool)
                          n203 = property on="Stop" class="Bool (strict)"("Value"=FALSE ("Stop")) -> ()  [unwired: 2 in, 2 out]
                          n204 = property on="StopAcq" class="Bool (strict)"("Value"=w343) -> ()  [unwired: 2 in, 2 out]
                        }
                      }
                      n205 = Request Deallocation(TRUE ("flag")) -> ()
                    }
                  }
                  n206 = Index Array "ITI"(array=w331, index=3) -> (element=w329:sgl)
                  n207 = Divide(x=w329, y=sgl 2.0) -> (x/y=w327:sgl)
                  n208 = Round Toward +Infinity(x=w327) -> (ceil(x): smallest int >= x=w326:sgl)
                  n209 = Wait (ms)(milliseconds to wait=w326) -> ()  [unwired: 1 out]
                  n210 = property on="Status" class="Str"("Value"="Writing files" ("String")) -> ()  [unwired: 2 in, 2 out]
                }
              }
              n211 = Or(x=w103, y=w102) -> (x .or. y?=w108:bool)
              "Odors:" <- w107
            }
          }
        }
        n212 = Index Array "#repeats"(array=w82, index=0) -> (element=w81:sgl)
        n213 = Equal?(x=w81, y=w86) -> (x = y?=w79:bool)
        n214 = Or(x=w79, y=w78) -> (x .or. y?=w87:bool)
      }
    }
    frame #2 {
      n215 = property on="ExpOrderRefnum" class="Ref (strict)"() -> ("Value"=w350:refnum<file>)  [unwired: 2 in, 2 out]
      n216 = property on="Status" class="Str"("Value"="Done!" ("Status")) -> ()  [unwired: 2 in, 2 out]
      n217 = property on="StopAcq" class="Bool (strict)"("Value"=TRUE ("StopAcq")) -> ()  [unwired: 2 in, 2 out]
      n218 = property on="IMAQ session" class="IMAQdx (strict)"() -> ("Value"=w348:refnum<k21>)  [unwired: 2 in, 2 out]
      n219 = call <vilib>:"IMAQdx Close Camera.vi"("Session In"=w348) -> ()  [unwired: 1 in, 10 out]
      n220 = Close File(refnum=w350) -> ()  [unwired: 1 in, 2 out]
    }
  }
